vi "Arduino Test.vi"() -> ()   [LabVIEW 2020]
uses:
  <vilib>/MakerHub/LINX/Public/Peripherals/Analog/Analog Read 1 Chan.vi
  <vilib>/MakerHub/LINX/Public/Peripherals/Analog/Analog Read N Chans.vi
  <vilib>/MakerHub/LINX/Private/Local IO/LinxAnalogRead.vi
  <vilib>/MakerHub/LINX/Public/Utilities/Check Channel.vi
  <vilib>/MakerHub/LINX/Public/Utilities/Open Serial.vi
  <vilib>/MakerHub/LINX/Private/Utilties/Generate Error.vi
  <vilib>/MakerHub/LINX/LMH-LINX.lvlib
  <vilib>/ptbypt/NI_PtbyPt.lvlib
panel:
  out "Voltage":dbl
  out "Hz":dbl format="%0.2f"
  out "Numeric":i32
  in  "Boolean":bool
  out "Device Name":string
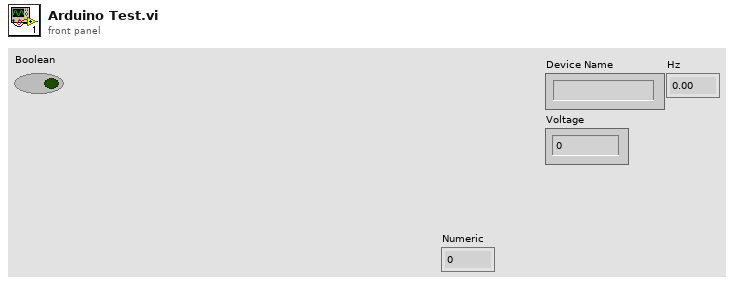
[diagram p1: front panel]
types:
  T1 = typedef "LMH-LINX.lvlib/LINX Ref.ctl" = cluster{"IO":T2, "Interface":T3, "LINX Device Config":T4}
  T2 = typedef "LMH-LINX.lvlib/Platform.ctl" = enum16{"Remote", "Local"}
  T3 = typedef "LMH-LINX.lvlib/Interface.ctl" = enum16{"Serial", "TCP"}
  T4 = typedef "LMH-LINX.lvlib/Device.lvlib/LINX Device Config.ctl" = cluster{"Interface":T3, "COM Port":refnum<visa-resource-name>, "TCP Configuration":T5, "Device Family":u8, "Device ID":u8, "Device Name":string, "TCP Ref":refnum<k5>, "Channels":T6}
  T5 = typedef "LMH-LINX.lvlib/Device.lvlib/TCP Config.ctl" = cluster{"IP Address":string, "Port":u16}
  T6 = typedef "LMH-LINX.lvlib/Channels.ctl" = cluster{"DI":u8[], "DO":u8[], "AI":u8[], "AO":u8[], "PWM":u8[], "QE":u8[], "UART":u8[], "I2C 2":u8[], "SPI":u8[], "CAN":u8[], "Servo":u8[], "AI Ref (V)":dbl, "AI Resolution (Bits)":u8, "AO Ref (V)":dbl, "AO Resolution (Bits)":u8}
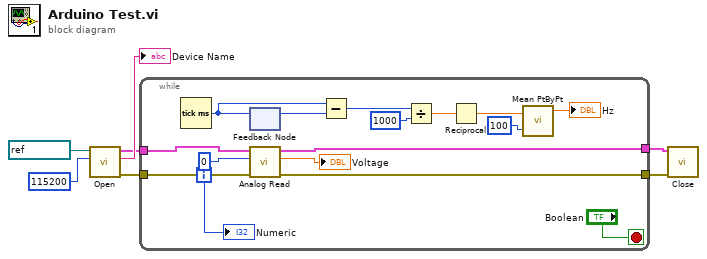
[diagram p0: block diagram]
diagram:
  n1 = call-poly <vilib>:"Open.vi"("Baud Rate Override"=u32 115200, "Serial Port"=refnum<visa-resource-name> "COM3") -> ("Error Out"=w4:errorcluster, "Device Name"=→"Device Name":string, "LINX Resource"=w5:T1)  [unwired: 7 in]
  n2 = while {
    tunnel: w5 -> [w23]
    tunnel: w4 -> [w12]
    tunnel: [w11] -> w2
    tunnel: [w10] -> w1
    i -> [w22]
    stop <- "Boolean" stop-if-true
    n3 = Tick Count (ms)() -> (millisecond timer value=w21:u32)
    n4 = feedback-in #1(w21) -> ()
    n5 = feedback #1() -> (w20:u32)  [unwired: 1 in]
    n6 = call-poly <vilib>:"Analog Read.vi"("Error In"=w12, "Analog Channel"=u8 0, "LINX Resource"=w23) -> ("Error Out"=w10:errorcluster, "Voltage"=→"Voltage":dbl, "LINX Resource"=w11:T1)  [unwired: 5 in, 1 out]
    n7 = Subtract(x=w21, y=w20) -> (x-y=w19:u32)
    n8 = Divide(x=w19, y=u32 1000) -> (x/y=w17:dbl)
    n9 = Reciprocal(x=w17) -> (1/x=w16:dbl)
    n10 = call <vilib>:"Mean PtByPt.vi"("x"=w16, "sample length"=100) -> ("mean"=→"Hz":dbl)  [unwired: 2 in, 1 out]
    "Numeric" <- w22
  }
  n11 = call <vilib>:"Close.vi"("Error In"=w1, "LINX Resource"=w2) -> ()  [unwired: 9 in, 1 out]
